vi "Read Max messagee size to send (octets).vi"(8 "error in (no error)":errorcluster, 11 "RawSocket Handler in":refnum<class "RawSocket Handler.lvclass">) -> (0 "error out":errorcluster, 2 "Max Messagre Size (octets)":u8, 3 "RawSocket Handler out":refnum<class "RawSocket Handler.lvclass">)   [LabVIEW 2020, in "wamplv.lvlib" / "RawSocket Handler.lvclass"]
uses:
  RawSocket Handler.lvclass
  RawSocket Handler.lvclass/RawSocket Handler.ctl
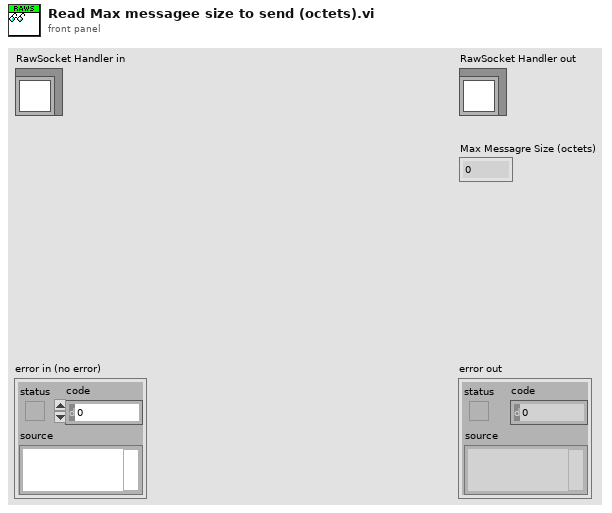
[diagram p1: front panel]
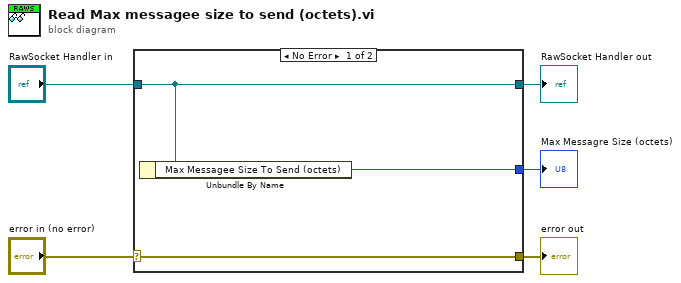
[diagram p0: block diagram]
diagram:
  n1 = case shown="No Error" "error in (no error)" {
    selector: "error in (no error)" -> [w8 w9]
    tunnel: [w8 w9] -> w4
    tunnel: [w7 w10] -> w2
    tunnel: "RawSocket Handler in" -> [w7 w10]
    tunnel: [w6 _] -> w1
    frame No Error {
      n2 = Unbundle By Name(w7) -> ("Max Messagee Size To Send (octets)"=w6:u8)
    }
    frame Error {
    }
  }
  "error out" <- w4
  "RawSocket Handler out" <- w2
  "Max Messagre Size (octets)" <- w1
